vi "GetCountsPerBin.vi"(11 "Counts until bin number":i32[](array[numeric])) -> (3 "Counts per Bin":dbl[](array[numeric]))   [LabVIEW 2013]
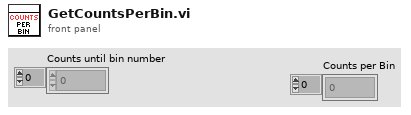
[diagram p1: front panel]
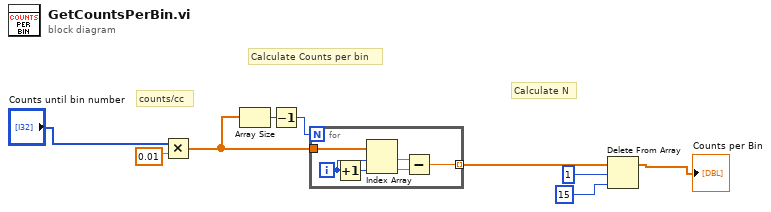
[diagram p0: block diagram]
diagram:
  # "counts/cc"
  # "Calculate N"
  # "Calculate Counts per bin"
  n1 = Multiply(x="Counts until bin number", y=0.01) -> (x*y=w3:dbl[])
  n2 = Array Size(array=w3) -> (size(s)=w9:i32)
  n3 = Decrement(x=w9) -> (x-1=w8:i32)
  n4 = for {
    N: w8 -> [_]
    tunnel: w3 -> [w15]
    tunnel: [w10] -> w7 mode=indexing
    i -> [w14]
    n5 = Increment(x=w14) -> (x+1=w13:i32)
    n6 = Index Array(array=w15, index #1=w14, index #2=w13) -> (element #1=w11:dbl, element #2=w12:dbl)
    n7 = Subtract(x=w11, y=w12) -> (x-y=w10:dbl)
  }
  n8 = Delete From Array(array=w7, length=1, index=15) -> (array with subset deleted=→"Counts per Bin":dbl[])  [unwired: 1 out]
